vi "Should Continue.vi"(8 "error in (no error)":errorcluster, 11 "TimedDirector in":refnum<class "TimedDirector.lvclass">) -> (0 "error out":errorcluster, 2 "Should Continue":bool, 3 "TimedDirector out":refnum<class "TimedDirector.lvclass">)   [LabVIEW 2023, in "HAF.lvlib" / "TimedDirector.lvclass"]
doc: "Returns true when the processing time has exceeded the duration."
uses:
  TimedDirector.lvclass
  TimedDirector.lvclass/TimedDirector.ctl
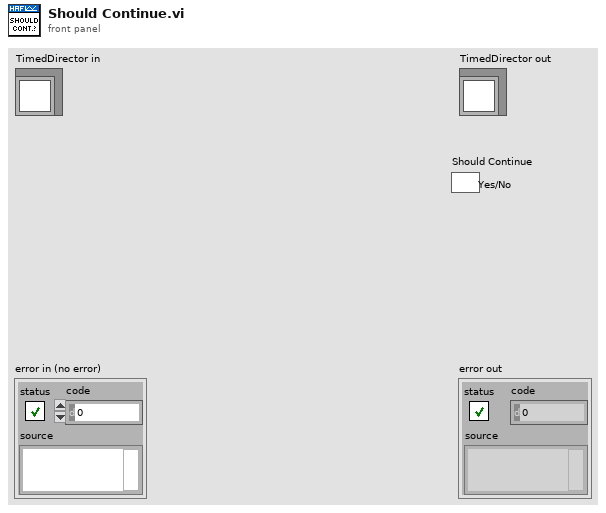
[diagram p1: front panel]
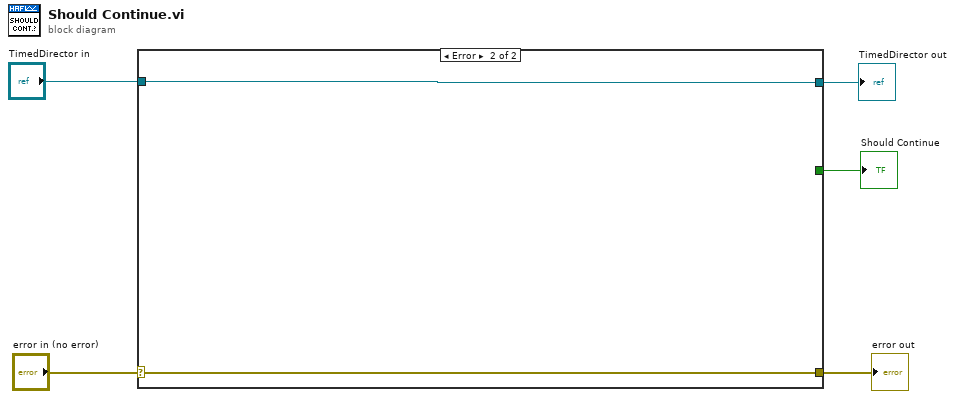
[diagram p0: block diagram]
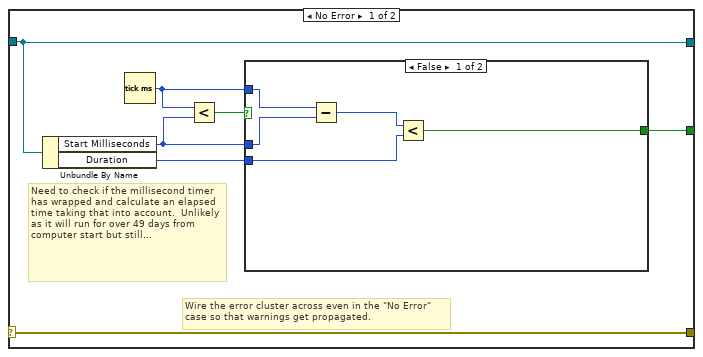
[diagram p2: hidden frame]
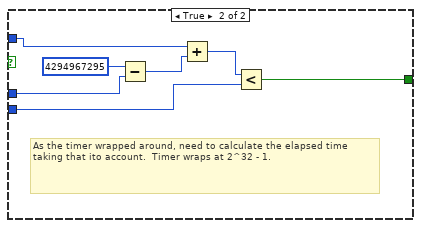
[diagram p3: hidden frame]
diagram:
  n1 = case shown="Error" "error in (no error)" {
    selector: "error in (no error)" -> [w12 w26]
    tunnel: [w12 w26] -> w4
    tunnel: [w11 w25] -> w2
    tunnel: "TimedDirector in" -> [w11 w25]
    tunnel: [w6 _] -> w1
    frame No Error {
      # "Need to check if the millisecond timer has wrapped and calculate an elapsed time taking that into account.  Unlikely as it will run for over 49 days from computer start but still..."
      # "Wire the error cluster across even in the \"No Error\"\ncase so that warnings get propagated."
      n2 = Unbundle By Name(w11) -> ("Start Milliseconds"=w8:u32, "Duration"=w7:u32)
      n3 = Tick Count (ms)() -> (millisecond timer value=w9:u32)
      n4 = Less?(x=w9, y=w8) -> (x < y?=w10:bool)
      n5 = case shown="False" w10 {
        tunnel: w9 -> [w17 w22]
        tunnel: w8 -> [w16 w23]
        tunnel: w7 -> [w14 w19]
        tunnel: [w13 w18] -> w6
        frame False {
          n6 = Subtract(x=w17, y=w16) -> (x-y=w15:u32)
          n7 = Less?(x=w15, y=w14) -> (x < y?=w13:bool)
        }
        frame True {
          # "As the timer wrapped around, need to calculate the elapsed time taking that ito account.  Timer wraps at 2^32 - 1."
          n8 = Subtract(x=u32 4294967295, y=w23) -> (x-y=w21:u32)
          n9 = Add(x=w22, y=w21) -> (x+y=w20:u32)
          n10 = Less?(x=w20, y=w19) -> (x < y?=w18:bool)
        }
      }
    }
    frame Error {
    }
  }
  "error out" <- w4
  "TimedDirector out" <- w2
  "Should Continue" <- w1
